vi "Amplitude and Phase Spectrum.vi"(3 "dt":dbl=1.0 format="%0.2f", 4 "unwrap phase (T)":bool=TRUE, 5 "Signal (V)":dbl[](array[numeric])) -> (0 "df":dbl format="%0.2f", 1 "Amp Spectrum Phase (radians)":dbl[](array[numeric]), 2 "Amp Spectrum Mag (Vrms)":dbl[](array[numeric]))   [LabVIEW 2014, in "NI_AALPro.lvlib"]
doc: "Computes the single-sided, scaled amplitude spectrum of a real-valued time-domain signal and returns the amplitude spectrum as magnitude and phase."
uses:
  NI_AALPro.lvlib
panel:
  # "Amplitude and\nPhase Spectrum"
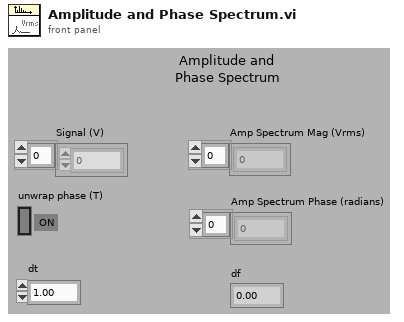
[diagram p1: front panel]
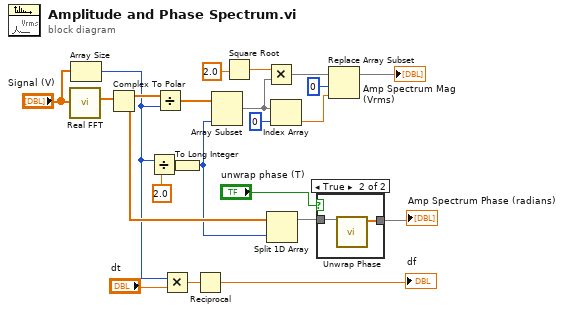
[diagram p0: block diagram]
diagram:
  n1 = call "Real FFT.vi"("X"="Signal (V)") -> ("FFT {X}"=w15:cdb[])  [unwired: 9 in, 1 out]
  n2 = Array Size(array="Signal (V)") -> (size(s)=w19:i32)
  n3 = Complex To Polar(r * e^(i*theta)=w15) -> (r=w23:dbl[], theta=w21:dbl[])
  n4 = Divide(x=w19, y=2.0) -> (x/y=w11:dbl)
  n5 = Divide(x=w23, y=w19) -> (x/y=w7:dbl[])
  n6 = Multiply(x=w19, y="dt") -> (x*y=w20:dbl)
  n7 = To Long Integer(number=w11) -> (32bit integer=w8:i32)
  n8 = Reciprocal(x=w20) -> (1/x=→"df":dbl)
  n9 = Array Subset(array=w7, length=w8) -> (w1:dbl[])  [unwired: 1 in]
  n10 = Square Root(x=2.0) -> (sqrt(x)=w3:dbl)
  n11 = Multiply(x=w3, y=w1) -> (x*y=w4:dbl[])
  n12 = Split 1D Array(array=w21, index=w8) -> (first subarray=w13:dbl[])  [unwired: 1 out]
  n13 = Index Array(array=w1, index=0) -> (element=w2:dbl)
  n14 = case shown="True" "unwrap phase (T)" {
    tunnel: w13 -> [w24 w26]
    tunnel: [w24 w25] -> w12
    frame False {
    }
    frame True {
      n15 = call "Unwrap Phase.vi"("Phase"=w26) -> ("Unwrapped Phase"=w25:dbl[])  [unwired: 9 in, 1 out]
    }
  }
  "Amp Spectrum Phase (radians)" <- w12
  n16 = Replace Array Subset(array=w4, new element=w2, index=0) -> (→"Amp Spectrum Mag (Vrms)":dbl[])
